vi "Speed_PI_Control.vi"(6 "analog voltage":dbl, 7 "Speed Ki":dbl(slide)=10.0 scale=1.0..10.0, 9 "Desired_Speed":dbl, 10 "Speed Kp":dbl(slide)=0.49679802955665026 scale=0.1..1.0, 11 "slope":dbl) -> (2 "Vm":dbl, 3 "Speed":dbl)   [LabVIEW 2012]
uses:
  <vilib>/Simulation/Implementation/Shared/SIMSCR Execution Mode.ctl
  <vilib>/Simulation/Scripting/Companion Diagram/SimConfigNode/SimParams.ctl
  <vilib>/Simulation/Scripting/Companion Diagram/SimConfigNode/_simSolvers.ctl
  <vilib>/Simulation/Param Hierarchy/Typedefs/SIMPH Param Control Actions.ctl
  <vilib>/Simulation/Implementation/Shared/SIM limit type.ctl
  <vilib>/Simulation/Implementation/Shared/NILVSim_ParamChanged.vi
  <vilib>/Simulation/SignalArithmetic/Implementation/NILVSim Gain.llb/SIM Gain (scalar).vi
  <vilib>/Simulation/Nonlinear/Implementation/NILVSim Saturation.llb/SIM Saturation (scalar).vi
  <vilib>/Simulation/ContinuousLinear/Implementation/NILVSim Integrator new.llb/SIM Integrator distributor (scalar).vi
  <vilib>/Simulation/ContinuousLinear/Implementation/NILVSim Integrator new.llb/SIM Integrator collector (scalar).vi
  <vilib>/Simulation/Implementation/Shared/NILVSim_Manager.vi
  <vilib>/Simulation/Implementation/Shared/NILVSim_FinalizeModel.vi
  <vilib>/Simulation/Implementation/Shared/SIM Unbundle Sim Info.vi
  <vilib>/Utility/error.llb/Clear Errors.vi
  <vilib>/Simulation/Implementation/Shared/NILVSim_GetModelError.vi
  <vilib>/Simulation/Implementation/Shared/SIM SimErrorHandler.vi
  <vilib>/Simulation/Implementation/Shared/SIM Bundle Sim Info.vi
  <vilib>/Simulation/Implementation/Shared/SIMSH Read Queue.vi
  <vilib>/Simulation/Implementation/Shared/NILVSim_Initialize.vi
  <vilib>/Simulation/Utility/Implementation/NILVSim Get Time and IsAcceptedStep.vi
  <vilib>/Simulation/Scripting/Companion Diagram/SimConfigNode/SimDog.xnode
  <vilib>/Simulation/Implementation/XNodeFramework/SimXNode/SimX.xnode
  <vilib>/Simulation/ContinuousLinear/Implementation/NILVSim Integrator new.llb/SIM Integrator (scalar).vi
  <vilib>/Simulation/Implementation/Shared/NI_SIM_Implementation.lvlib
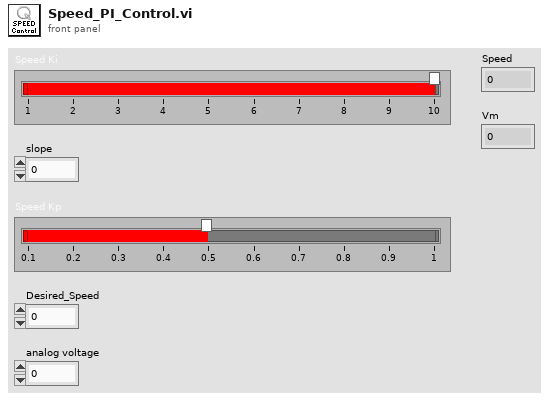
[diagram p1: front panel]
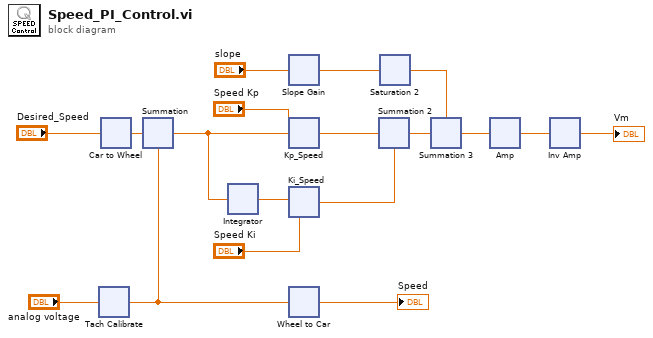
[diagram p0: block diagram]
diagram:
  n1 = xnode "Tach Calibrate"("input"="analog voltage") -> ("output"=w14:dbl)  [unwired: 3 in]
  n2 = xnode "Car to Wheel"("input"="Desired_Speed") -> ("output"=w13:dbl)  [unwired: 3 in]
  n3 = xnode ("Summation")("Operand1"=w13, "Operand2"=w14) -> ("Result"=w5:dbl)
  n4 = xnode "Integrator"("input"=w5) -> ("output"=w6:dbl)  [unwired: 9 in, 2 out]
  n5 = xnode "Slope Gain"("input"="slope") -> ("output"=w9:dbl)  [unwired: 3 in]
  n6 = xnode ("Kp_Speed")("gain"="Speed Kp", "input"=w5) -> ("output"=w4:dbl)  [unwired: 2 in]
  n7 = xnode ("Ki_Speed")("gain"="Speed Ki", "input"=w6) -> ("output"=w7:dbl)  [unwired: 2 in]
  n8 = xnode "Wheel to Car"("input"=w14) -> ("output"=→"Speed":dbl)  [unwired: 3 in]
  n9 = xnode ("Summation 2")("Operand1"=w4, "Operand2"=w7) -> ("Result"=w8:dbl)
  n10 = xnode ("Saturation 2")("input"=w9) -> ("output"=w10:dbl)  [unwired: 4 in]
  n11 = xnode ("Summation 3")("Operand1"=w10, "Operand2"=w8) -> ("Result"=w2:dbl)
  n12 = xnode "Amp"("input"=w2) -> ("output"=w3:dbl)  [unwired: 4 in]
  n13 = xnode "Inv Amp"("input"=w3) -> ("output"=→"Vm":dbl)  [unwired: 3 in]
